vi "ControlVoltage_NICard.vi"() -> ()   [LabVIEW 2017]
uses:
  <vilib>/Analysis/baseanly.llb/Mean (DBL).vi
  VoltageQueue_Global.vi
  MessageQueue/QueueOperations/Enqueue Message (Single).vi
  PowerMeter_Measurement.vi
  MessageQueue/MessageQueue.lvlib
  <vilib>/Analysis/NI_AALBase.lvlib
panel:
  in  "dV":dbl=0.01 format="%#_13g"
  out "Stoped":bool=TRUE
  in  "Controler time (ms)":u32
  out "mean":dbl format="%.3p"
  out "standard deviation":dbl format="%.3p"
  in  "Power (W)":dbl format="%#_6p"
  out "Past Power List":dbl[](array[numeric])
  in  "Initial Voltage":dbl
  out "XY Graph":cluster{dbl[], dbl[]}(graph)
  in  "dt (ms)":u32=10
  in  "Plot Length":i32=10000
  in  "stop":bool
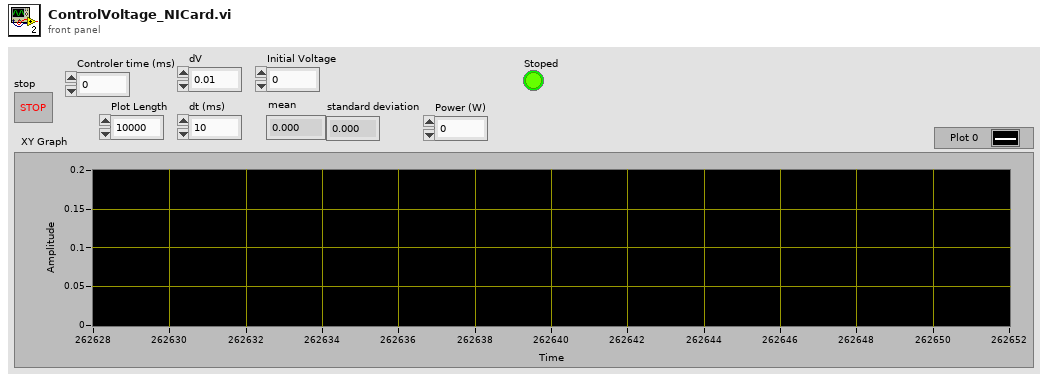
[diagram p1: front panel]
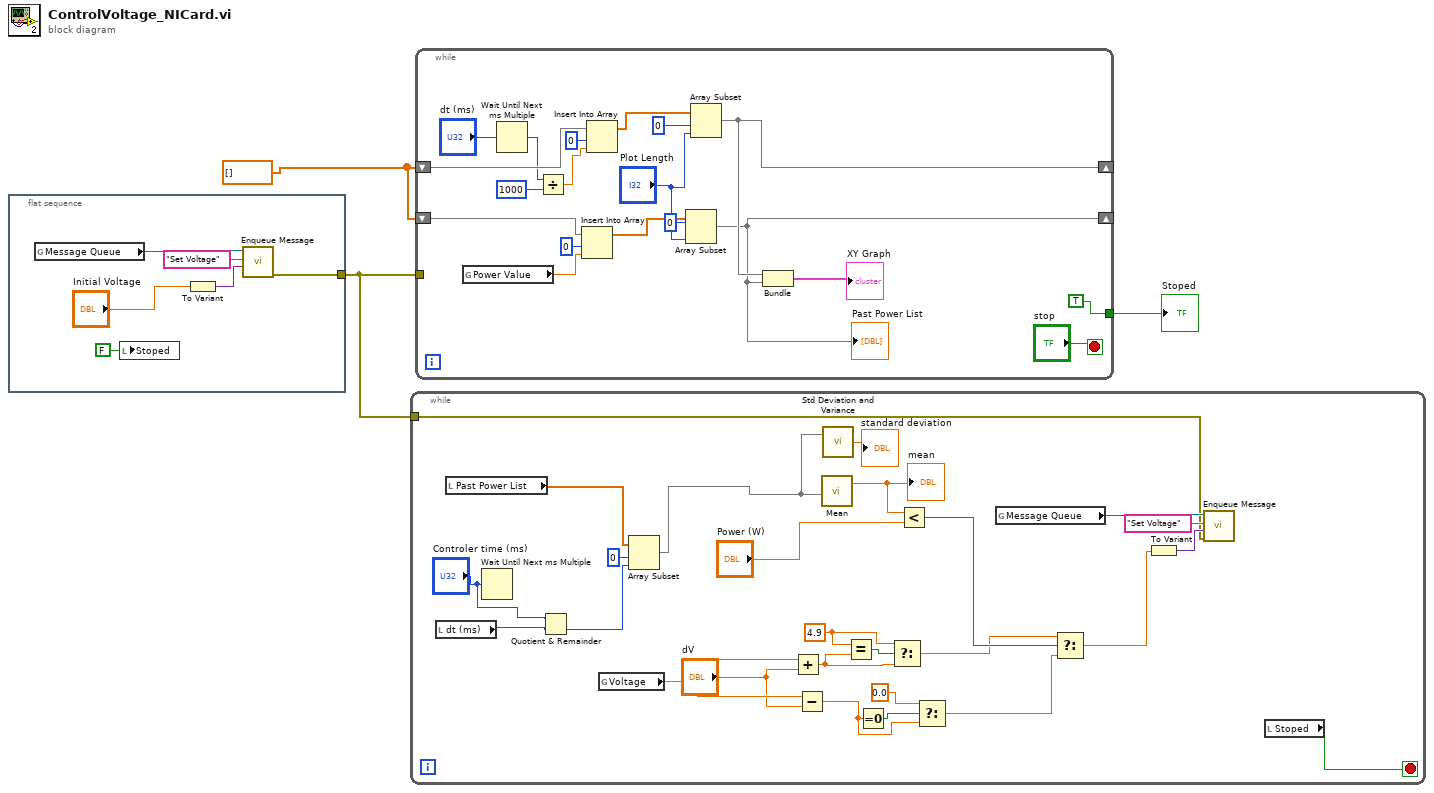
[diagram p0: block diagram]
diagram:
  w3 = dbl[] []
  n1 = flat-sequence {
    tunnel: [w4] -> w1
    frame #0 {
      n2 = global read "VoltageQueue_Global.vi" "Message Queue"() -> (w9:refnum<queue>)
      n3 = local write "Stoped"(FALSE ("Stoped")) -> ()
      n4 = To Variant(anything="Initial Voltage") -> (Variant=w8:variant)
      n5 = call-poly "Enqueue Message.vi"("Message Data"=w8, "Message"="Set Voltage", "Message Queue"=w9) -> ("error out"=w4:errorcluster)  [unwired: 7 in, 1 out]
    }
  }
  n6 = while {
    tunnel: w1 -> [w16]
    stop <- w17 stop-if-true
    w20 = 4.9 ("y")
    n7 = local read "dt (ms)"() -> (w14:u32)
    n8 = local read "Past Power List"() -> (w11:dbl[])
    n9 = Wait Until Next ms Multiple(millisecond multiple="Controler time (ms)") -> ()  [unwired: 1 out]
    n10 = Quotient & Remainder(x="Controler time (ms)", y=w14) -> (floor(x/y)=w12:u32)  [unwired: 1 out]
    n11 = global read "VoltageQueue_Global.vi" "Voltage"() -> (w29:dbl)
    n12 = Array Subset(array=w11, index=0, length=w12) -> (w10:dbl[])
    n13 = Add(x=w29, y="dV") -> (x+y=w19:dbl)
    n14 = Subtract(x=w29, y="dV") -> (x-y=w25:dbl)
    n15 = call-poly <vilib>:"Mean.vi"("X"=w10) -> ("mean"=w34:dbl)  [unwired: 1 out]
    "mean" <- w34
    n16 = call <vilib>:"Std Deviation and Variance.vi"("X"=w10) -> ("standard deviation"=→"standard deviation":dbl)  [unwired: 1 in, 2 out]
    n17 = Equal?(x=w20, y=w19) -> (x = y?=w22:bool)
    n18 = Equal To 0?(x=w25) -> (x = 0?=w26:bool)
    n19 = Select(t=w20, s=w22, f=w19) -> (s? t:f=w21:dbl)
    n20 = Less?(x=w34, y="Power (W)") -> (x < y?=w35:bool)
    n21 = Select(t=0.0 ("y"), s=w26, f=w25) -> (s? t:f=w23:dbl)
    n22 = global read "VoltageQueue_Global.vi" "Message Queue"() -> (w32:refnum<queue>)
    n23 = Select(t=w21, s=w35, f=w23) -> (s? t:f=w27:dbl)
    n24 = To Variant(anything=w27) -> (Variant=w31:variant)
    n25 = call-poly "Enqueue Message.vi"("error in (no error)"=w16, "Message Data"=w31, "Message"="Set Voltage", "Message Queue"=w32) -> ()  [unwired: 6 in, 2 out]
    n26 = local read "Stoped"() -> (w17:bool)
  }
  n27 = while {
    shift-right: [w37] -> _
    shift-left: w3 -> [w41]
    shift-right: [w48] -> _
    shift-left: w3 -> [w49]
    tunnel: [TRUE] -> w2
    tunnel: w1 -> [_]
    stop <- "stop" stop-if-true
    n28 = global read "PowerMeter_Measurement.vi" "Power Value"() -> (w43:dbl)
    n29 = Wait Until Next ms Multiple(millisecond multiple="dt (ms)") -> (millisecond timer value=w45:u32)
    n30 = Divide(x=w45, y=u32 1000) -> (x/y=w44:dbl)
    n31 = Insert Into Array(array=w41, index=0, new element=w43) -> (w40:dbl[])
    n32 = Insert Into Array(array=w49, index=0, new element=w44) -> (w52:dbl[])
    n33 = Array Subset(array=w40, index=0, length="Plot Length") -> (w37:dbl[])
    "Past Power List" <- w37
    n34 = Array Subset(array=w52, index=0, length="Plot Length") -> (w48:dbl[])
    n35 = Bundle(w48, w37) -> (→"XY Graph":cluster{dbl[], dbl[]})  [unwired: 1 in]
  }
  "Stoped" <- w2
